vi "CostFunction MSE.vi"(9 "Data points":sgl, 10 "Label (expected output":sgl, 11 "Output":sgl) -> (3 "x/y":sgl)   [LabVIEW 2020]
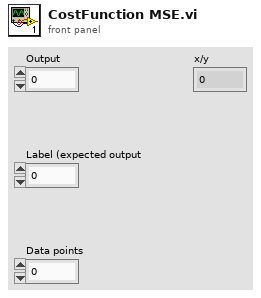
[diagram p1: front panel]
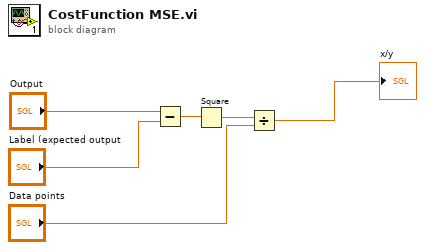
[diagram p0: block diagram]
diagram:
  n1 = Subtract(x="Output", y="Label (expected output") -> (x-y=w3:sgl)
  n2 = Square(x=w3) -> (x^2=w4:sgl)
  n3 = Divide(x=w4, y="Data points") -> (x/y=→"x/y":sgl)
